vi "Call DQMH Is Broadcast VI.vi"(8 "error in":errorcluster, 11 "Request VI in":refnum<vi>) -> (0 "error out":errorcluster, 2 "Is Broadcast":bool, 3 "Request VI out":refnum<vi>)   [LabVIEW 2017, in "Open DQMH Request Message Diagram.lvlib"]
doc: "Call is Broadcast VI.\n\nBSD 3-Clause License\n\nCopyright (c) 2022, Neosoft Technologies Inc\nAll rights reserved.\n\nRedistribution and use in source and binary forms, with or without\nmodification, are permitted provided that the following conditions are met:\n\n1. Redistributions of source code must retain the above copyright notice, this\n list of conditions and the following disclaimer.\n\n2. Redistributions in binary form must reproduce the above copyright notice,\n this list of conditions and the following disclaimer in the documentation\n and/or other materials provided with the distribution.\n\n3. Neither the name of the copyright holder nor the names of its\n contributors may be used to endorse or promote products derived from\n this software without specific prior written permission.\n\nTHIS SOFTWARE IS PROVIDED BY THE COPYRIGHT HOLDERS AND CONTRIBUTORS \"AS IS\"\nAND ANY EXPRESS OR IMPLIED WARRANTIES, INCLUDING, BUT NOT LIMITED TO, THE\nIMPLIED WARRANTIES OF MERCHANTABILITY AND FITNESS FOR A PARTICULAR PURPOSE ARE\nDISCLAIMED. IN NO EVENT SHALL THE COPYRIGHT HOLDER OR CONTRIBUTORS BE LIABLE\nFOR ANY DIRECT, INDIRECT, INCIDENTAL, SPECIAL, EXEMPLARY, OR CONSEQUENTIAL\nDAMAGES (INCLUDING, BUT NOT LIMITED TO, PROCUREMENT OF SUBSTITUTE GOODS OR\nSERVICES; LOSS OF USE, DATA, OR PROFITS; OR BUSINESS INTERRUPTION) HOWEVER\nCAUSED AND ON ANY THEORY OF LIABILITY, WHETHER IN CONTRACT, STRICT LIABILITY,\nOR TORT (INCLUDING NEGLIGENCE OR OTHERWISE) ARISING IN ANY WAY OUT OF THE USE\nOF THIS SOFTWARE, EVEN IF ADVISED OF THE POSSIBILITY OF SUCH DAMAGE."
uses:
  Open DQMH Request Message Diagram.lvlib
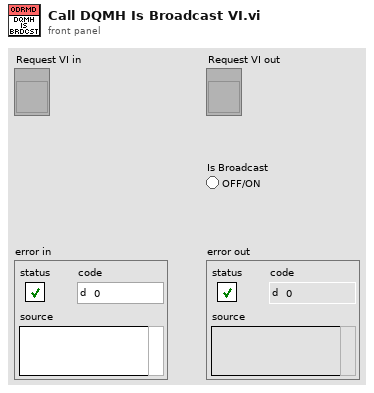
[diagram p1: front panel]
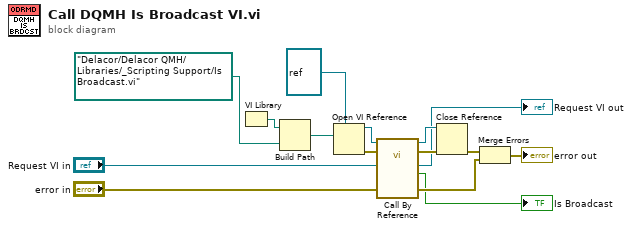
[diagram p0: block diagram]
diagram:
  n1 = VI Library() -> (path=w7:path)
  n2 = Build Path(base path=w7, name or relative path=path "Delacor/Delacor QMH/Libraries/_Scripting Support/Is Broadcast.vi") -> (appended path=w6:path)
  n3 = Open VI Reference(type specifier VI Refnum (for type only)=refnum<vi> refnum, vi path=w6) -> (vi reference=w9:refnum<vi>, error out=w12:errorcluster)  [unwired: 4 in]
  n4 = call-by-ref "?"(reference=w9, error in=w12, 8:"error in (no error)"="error in", "Request VI in"="Request VI in") -> (reference out=w8:refnum<vi>, error out=w15:errorcluster, 0:"error out"=w14:errorcluster, "Is Broadcast"=→"Is Broadcast":bool, "Request VI out"=→"Request VI out":refnum<vi>)  [unwired: 7 in]
  n5 = Close Reference(reference=w8, error in (no error)=w15) -> (error out=w13:errorcluster)
  n6 = Merge Errors(w13, w14) -> (→"error out":errorcluster)
